vi "Shifting button.vi"(9 "ShiftDownButton":bool, 10 "ShiftUpButton":bool, 11 "AutoButton":bool) -> ()   [LabVIEW 2015]
uses:
  Robot Global Data.vi
panel:
  in  "GearButton":bool
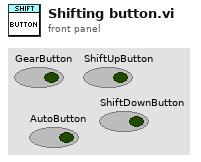
[diagram p1: front panel]
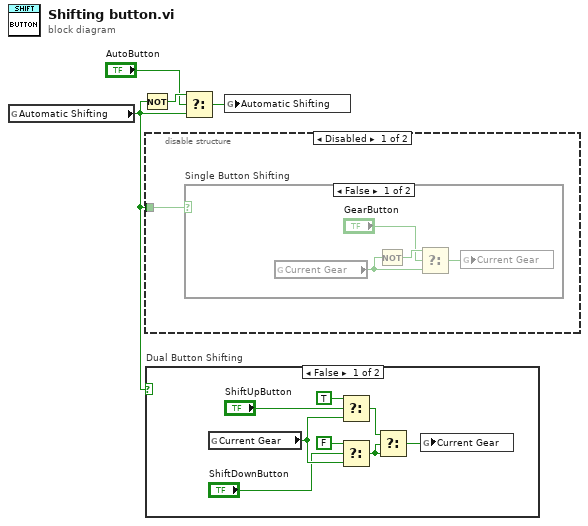
[diagram p0: block diagram]
diagram:
  n1 = global read "Robot Global Data.vi" "Automatic Shifting"() -> (w1:bool)
  n2 = Not(x=w1) -> (.not. x?=w3:bool)
  n3 = disable-structure shown="Disabled" {
    disable-tunnel: w1 -> [w5 _]
    frame Disabled {
      n4 = case "Single Button Shifting" shown="False" w5 {
        frame False {
          n5 = global read "Robot Global Data.vi" "Current Gear"() -> (w6:bool)
          n6 = Not(x=w6) -> (.not. x?=w9:bool)
          n7 = Select(t=w9, s="GearButton", f=w6) -> (s? t:f=w8:bool)
          n8 = global write "Robot Global Data.vi" "Current Gear"(w8) -> ()
        }
        frame True {
        }
      }
    }
    frame Enabled {
    }
  }
  n9 = case "Dual Button Shifting" shown="False" w1 {
    frame False {
      n10 = global read "Robot Global Data.vi" "Current Gear"() -> (w14:bool)
      n11 = Select(t=TRUE, s="ShiftUpButton", f=w14) -> (s? t:f=w16:bool)
      n12 = Select(t=FALSE, s="ShiftDownButton", f=w14) -> (s? t:f=w15:bool)
      n13 = Select(t=w16, s=w15, f=w15) -> (s? t:f=w17:bool)
      n14 = global write "Robot Global Data.vi" "Current Gear"(w17) -> ()
    }
    frame True {
    }
  }
  n15 = Select(t=w3, s="AutoButton", f=w1) -> (s? t:f=w4:bool)
  n16 = global write "Robot Global Data.vi" "Automatic Shifting"(w4) -> ()
